vi "习4.7.vi"() -> ()   [LabVIEW 2017]
panel:
  out "猜测值":dbl
  out "随机的数":u64
  out "猜测次数":i32
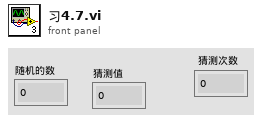
[diagram p1: front panel]
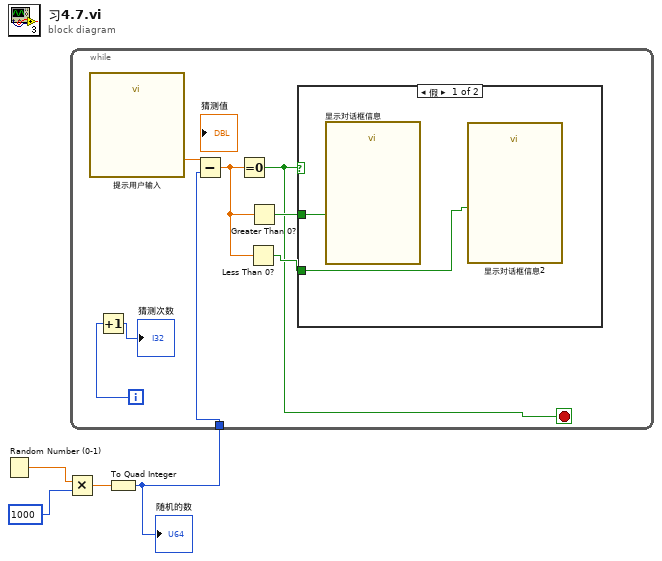
[diagram p0: block diagram]
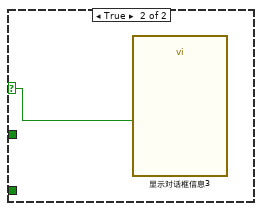
[diagram p2: hidden frame]
diagram:
  n1 = Random Number (0-1)() -> (number: 0 to 1=w4:dbl)
  n2 = Multiply(x=w4, y=1000) -> (x*y=w2:dbl)
  n3 = To Quad Integer(1:w2) -> (0:w1:i64)
  "随机的数" <- w1
  n4 = while {
    tunnel: w1 -> [w10]
    i -> [w12]
    stop <- w6 stop-if-true
    n5 = call "提示用户输入"() -> ("请在1-1000猜"=w5:dbl)  [unwired: 17 in, 2 out]
    n6 = Increment(x=w12) -> (x+1=→"猜测次数":i32)
    n7 = Subtract(x=w5, y=w10) -> (x-y=w8:dbl)
    n8 = Equal To 0?(x=w8) -> (x = 0?=w6:bool)
    n9 = Less Than 0?(x=w8) -> (x < 0?=w7:bool)
    n10 = Greater Than 0?(x=w8) -> (x > 0?=w9:bool)
    n11 = case shown="假" w6 {
      selector: w6 -> [_ w15]
      tunnel: w9 -> [w14 _]
      tunnel: w7 -> [w13 _]
      frame False {
        n12 = call "显示对话框信息"("Enable"=w14) -> ()  [unwired: 9 in, 2 out]
        n13 = call "显示对话框信息2"("Enable"=w13) -> ()  [unwired: 9 in, 2 out]
      }
      frame True {
        n14 = call "显示对话框信息3"("Enable"=w15) -> ()  [unwired: 9 in, 2 out]
      }
    }
  }
